vi "closeKuka.vi"(8 "错误输入（无错误）":errorcluster, 11 "TCP网络连接输入":refnum<k5>) -> ()   [LabVIEW 2015, in "labOpenShowVar.lvlib"]
uses:
  labOpenShowVar.lvlib
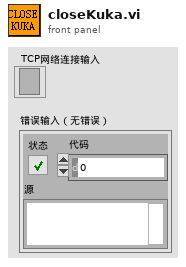
[diagram p1: front panel]
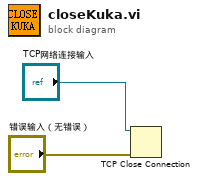
[diagram p0: block diagram]
diagram:
  n1 = TCP Close Connection(connection ID="TCP网络连接输入", error in (no error)="错误输入（无错误）") -> ()  [unwired: 1 in, 2 out]
